vi "Add Run.vi"(8 "error in (no error)":errorcluster, 9 "Number of repetitions":u32, 10 "Run Instance":refnum<class "Run Instance.lvclass">, 11 "Schedule in":refnum<class "Schedule.lvclass">) -> (0 "error out":errorcluster, 3 "Schedule out":refnum<class "Schedule.lvclass">)   [LabVIEW 2020, in "CIRCUS_uServices.lvlib" / "Run Utilities.lvlib" / "Schedule.lvclass"]
doc: "Vi for adding new Run Instance into the schedule. It appends the value to the existing array"
uses:
  Schedule.lvclass
  Run Instance/Run Instance.lvclass
  Cell/Schedule Cell.lvclass
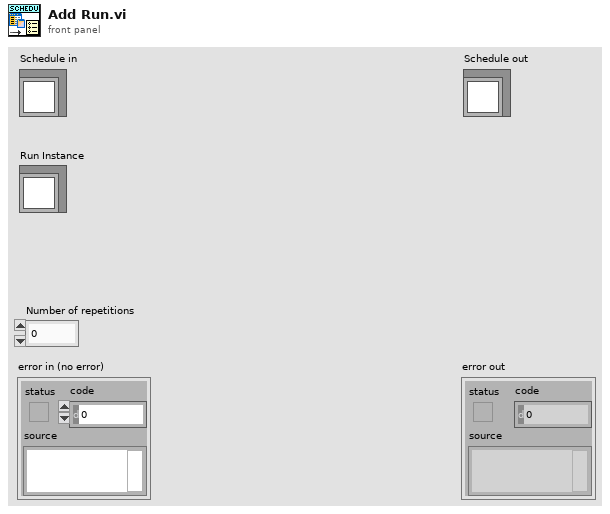
[diagram p1: front panel]
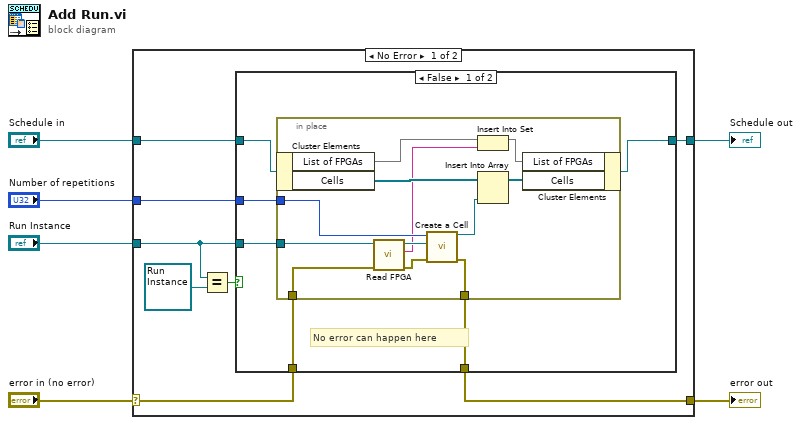
[diagram p0: block diagram]
diagram:
  n1 = case shown="No Error" "error in (no error)" {
    selector: "error in (no error)" -> [w8 w36]
    tunnel: [w7 w36] -> w5
    tunnel: [w13 w35] -> w3
    tunnel: "Schedule in" -> [w14 w35]
    tunnel: "Run Instance" -> [w11 _]
    tunnel: "Number of repetitions" -> [w12 _]
    frame No Error {
      n2 = Equal?(x=w11, y=refnum<class "Run Instance.lvclass"> refnum ("Run Instance")) -> (x = y?=w9:bool)
      n3 = case shown="False" w9 {
        tunnel: w14 -> [w16 w34]
        tunnel: [w15 w34] -> w13
        tunnel: w12 -> [w18 _]
        tunnel: w11 -> [w17 _]
        tunnel: w8 -> [w20 w33]
        tunnel: [w19 w33] -> w7
        frame False {
          # "No error can happen here"
          n4 = in-place {
            in-place-border: w20 -> [w25]
            in-place-border: [w31] -> w19
            in-place-border: w18 -> [w30]
            in-place-border: w17 -> [w27]
            n5 = in-place-cluster #1(w16) -> ("List of FPGAs"=w23:set{string}, "Cells"=w28:refnum<class "Schedule Cell.lvclass">[])
            n6 = call-dynamic "Read FPGA.vi"("error in (no error)"=w25, "Run Instance in"=w27) -> ("error out"=w24:errorcluster, "FPGA Name"=w21:string, "Run Instance out"=w26:refnum<class "Run Instance.lvclass">)  [unwired: 7 in]
            n7 = call "Create a Cell.vi"("error in (no error)"=w24, "Run Instance"=w26, "Repetitions"=w30) -> ("error out"=w31:errorcluster, "Schedule Cell out"=w32:refnum<class "Schedule Cell.lvclass">)  [unwired: 7 in]
            n8 = Insert Into Set(10:w21, 11:w23) -> (3:w22:set{string})  [unwired: 1 out]
            n9 = Insert Into Array(array=w28, new element=w32) -> (w29:refnum<class "Schedule Cell.lvclass">[])  [unwired: 1 in]
            n10 = in-place-cluster #1("List of FPGAs"=w22, "Cells"=w29) -> (w15:refnum<class "Schedule.lvclass">)
          }
        }
        frame True {
          # "Run Instance is empty, do nothing"
        }
      }
    }
    frame Error {
    }
  }
  "error out" <- w5
  "Schedule out" <- w3
